vi "Constants.vi"(11 "error in":errorcluster) -> (4 "Source path":path, 6 "Drona ini file path":path, 15 "error out":errorcluster)   [LabVIEW 2016, in "Drona.lvlib"]
doc: "Gives out required paths"
uses:
  Drona.lvlib
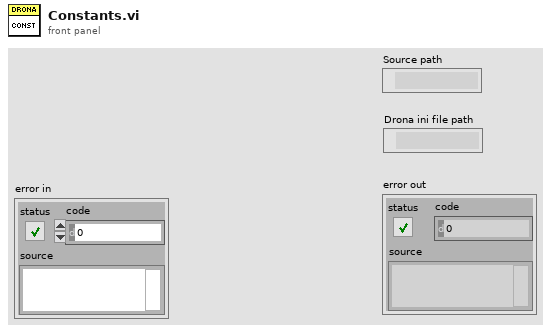
[diagram p1: front panel]
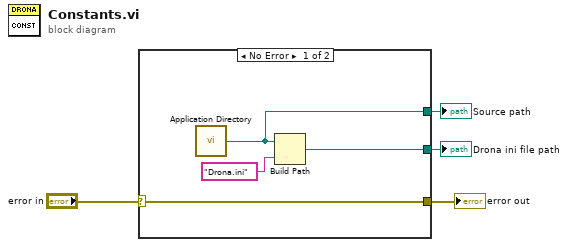
[diagram p0: block diagram]
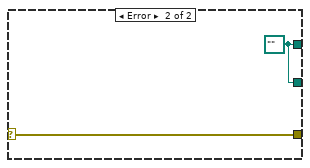
[diagram p2: hidden frame]
diagram:
  n1 = case shown="No Error" "error in" {
    selector: "error in" -> [w5 w10]
    tunnel: [w7 w9] -> w2
    tunnel: [w6 w9] -> w1
    tunnel: [w5 w10] -> w3
    frame No Error {
      n2 = call <vilib>:"Application Directory.vi"() -> ("Application Directory"=w6:path)
      n3 = Build Path(base path=w6, name or relative path="Drona.ini") -> (appended path=w7:path)
    }
    frame Error {
      w9 = path "" ("Application Directory")
    }
  }
  "error out" <- w3
  "Drona ini file path" <- w2
  "Source path" <- w1
